vi "Device Settings Session.vi"(2 "Error In":errorcluster, 3 "Type":enum16{"Set Settings", "Get Settings"}(ring)=enum."Get Settings") -> (0 "Error Out":errorcluster, 1 "Device Settings":T1={"Device Type"="", "Device Name"="", "DAQmx Name"="Dev1", "Terminal Wiring"=10106} {"Terminal Wiring" items=["Default"=-1, "RSE"=10083, "NRSE"=10078, "Differential"=10106, "Pseudodifferential"=12529]})   [LabVIEW 2019]
uses:
  Controls/Device Settings.ctl
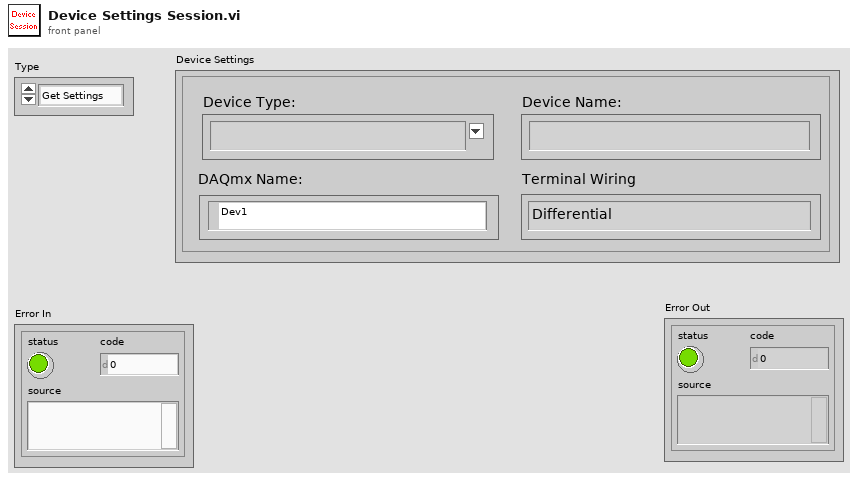
[diagram p1: front panel]
types:
  T1 = typedef "Device Settings.ctl" = cluster{"Device Type":string, "Device Name":string, "DAQmx Name":tag, "Terminal Wiring":i32}
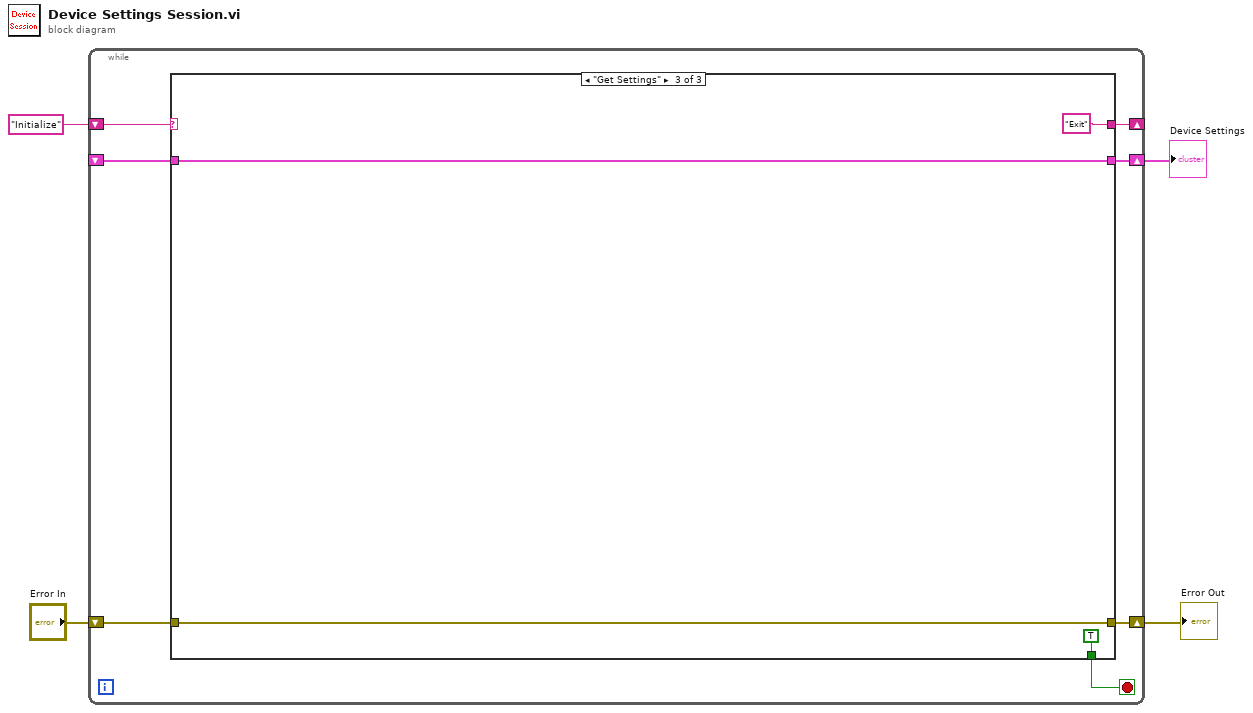
[diagram p0: block diagram]
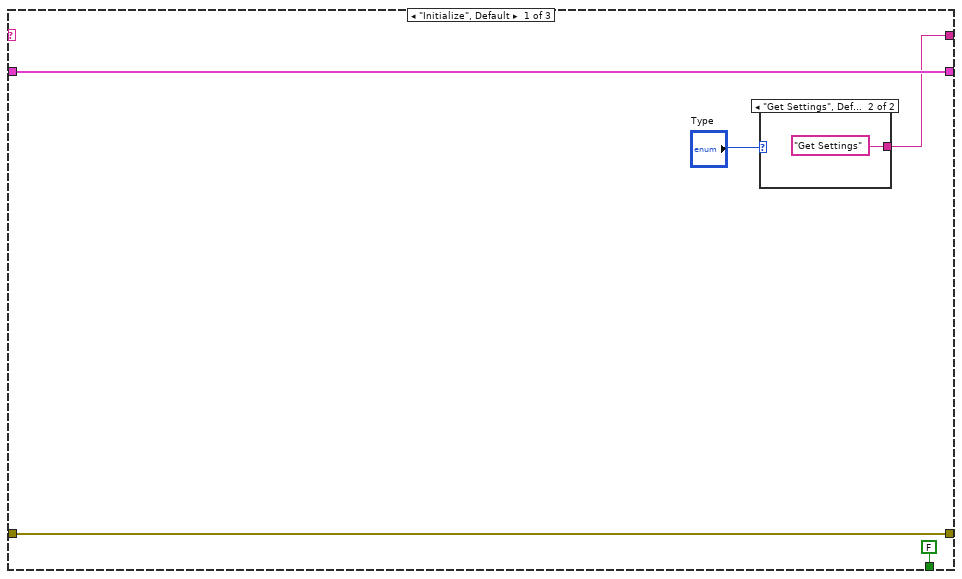
[diagram p2: hidden frame]
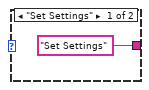
[diagram p3: hidden frame]
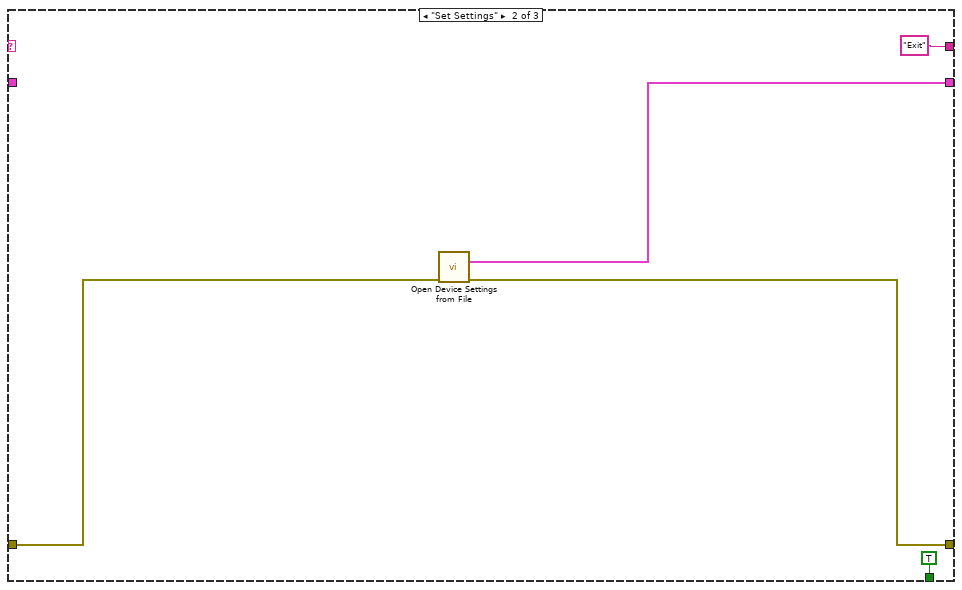
[diagram p4: hidden frame]
diagram:
  n1 = while {
    shift-right: [w6] -> _
    shift-left: "Initialize" ("key") -> [w11]
    shift-right: [w7] -> w1
    shift-left: _ -> [w10]
    shift-right: [w8] -> w2
    shift-left: "Error In" -> [w9]
    stop <- w5 stop-if-true
    n2 = case shown="\"Get Settings\"" w11 {
      tunnel: w10 -> [w14 _ w24]
      tunnel: w9 -> [w15 w21 w25]
      tunnel: [w15 w20 w25] -> w8
      tunnel: [w14 w19 w24] -> w7
      tunnel: [w12 "Exit" ("key") "Exit" ("key")] -> w6
      tunnel: [FALSE TRUE TRUE] -> w5
      frame "Initialize", Default {
        n3 = case shown="\"Get Settings\", Default" "Type" {
          tunnel: ["Set Settings" ("key") "Get Settings" ("key")] -> w12
          frame "Set Settings" {
          }
          frame "Get Settings", Default {
          }
        }
      }
      frame "Set Settings" {
        n4 = call "Open Device Settings from File.vi"("Error In"=w21) -> ("Device Settings"=w19:T1, "Error Out"=w20:errorcluster)  [unwired: 13 in]
      }
      frame "Get Settings" {
      }
    }
  }
  "Error Out" <- w2
  "Device Settings" <- w1
